vi "AlliGator Save IRFs & Fit Data (Map) HDF5 File v0.4.vi"(0 "File Path":path, 5 "IRFs & Fit Data Map v2":T12 {"Fit Options: Decay Preprocessing Parameters"."# Folds" min=1}, 7 "Decay Fit Options & Parameters":T1 {"Fit Options"."Offset Resolution" min=0.0; "Fit Options"."Period" min=0.0; "Fit Options"."Min Decay Percentile" min=0.0 max=1.0; "Fit Options"."Max Decay Percentile" min=0.0 max=100.0; "Fit Parameter Constraints"."Max Value" format="%#.3g"; "Fit Parameter Constraints"."Min Value" format="%#.3g"}, 9 "Software + Version":string, 11 "Error In":errorcluster, 12 "[Multiple Decays Fit Parameters SDV]":dbl[][](array[numeric])) -> (4 "File Path out":path, 14 "Time (s)":dbl, 15 "Error Out":errorcluster)   [LabVIEW 2021, in "AlliGator Decay Fit Parameter Map.lvlib"]
doc: "Saves Decay Fit Parameter Map and associated metadata to an HDF5 file."
uses:
  AlliGator Decay Fit Parameter Map.lvlib
  AlliGator IRFs & Fit Data v2.ctl
  Fits/IRF(X)PSED/Decay Fit Parameters & Derived Quantities List v2.ctl
  Decay Analysis/Decay Preprocessing/AlliGator Decay Preprocessing Parameters.ctl
  Graphs/XY Graph/XY Graph Plot Shift Parameters.ctl
  Graphs/XY Graph/XY Graph Plot Shift Method.ctl
  AlliGator Decay Fit Options & Parameters v2.ctl
  Fits/IRF(X)PSED/Decay Fit Options v2.ctl
  Fits/Decay Convolution/Decay Model.ctl
  Fits/Residual Type.ctl
  Fits/IRF(X)PSED/Fit Weights Type.ctl
  Fits/Non-linear Fitting Method v2.ctl
  Fits/Fit Calculation Method.ctl
  Fits/Non-linear Fitting Algorithm.ctl
  Decay Analysis/Decay Fit/AlliGator Decay Fit Parameter Constraints 2.ctl
  Fits/IRF(X)PSED/Decay Fit Parameters In List.ctl
  Fits/IRF(X)PSED/MLE Baseline Offset Type.ctl
  <vilib>/addons/h5labview2/file/H5Fmode.ctl
  Globals, Variables, Constants/AlliGator Variables List.ctl
  <vilib>/addons/h5labview2/base/lib_path.vi
  <vilib>/addons/h5labview2/base/H5Equery.vi
  Variant/Variant to Data/Variant to String.vi
  <vilib>/addons/h5labview2/dataset/H5Dwrite.llb/H5Dwrite.xnode
  <vilib>/addons/h5labview2/base/hid_t.ctl
  <vilib>/addons/h5labview2/file/H5F.lvlib
  <vilib>/addons/h5labview2/group/H5G.lvlib
  Time/Time.lvlib
  Utilities/Utilities.lvlib
  Strings/Strings.lvlib
  Globals, Variables, Constants/AlliGator Globals, Variables & Constants.lvlib
  Variant/Variant to Data/Variant to Data.lvlib
  Fits/Fits.lvlib
  Graphs/XY Graph/XY Graph Add-Ons.lvlib
  Decay Analysis/Decay Preprocessing/AlliGator Decay Preprocessing.lvlib
  Decay Analysis/Decay Fit/AlliGator Decay Fit.lvlib
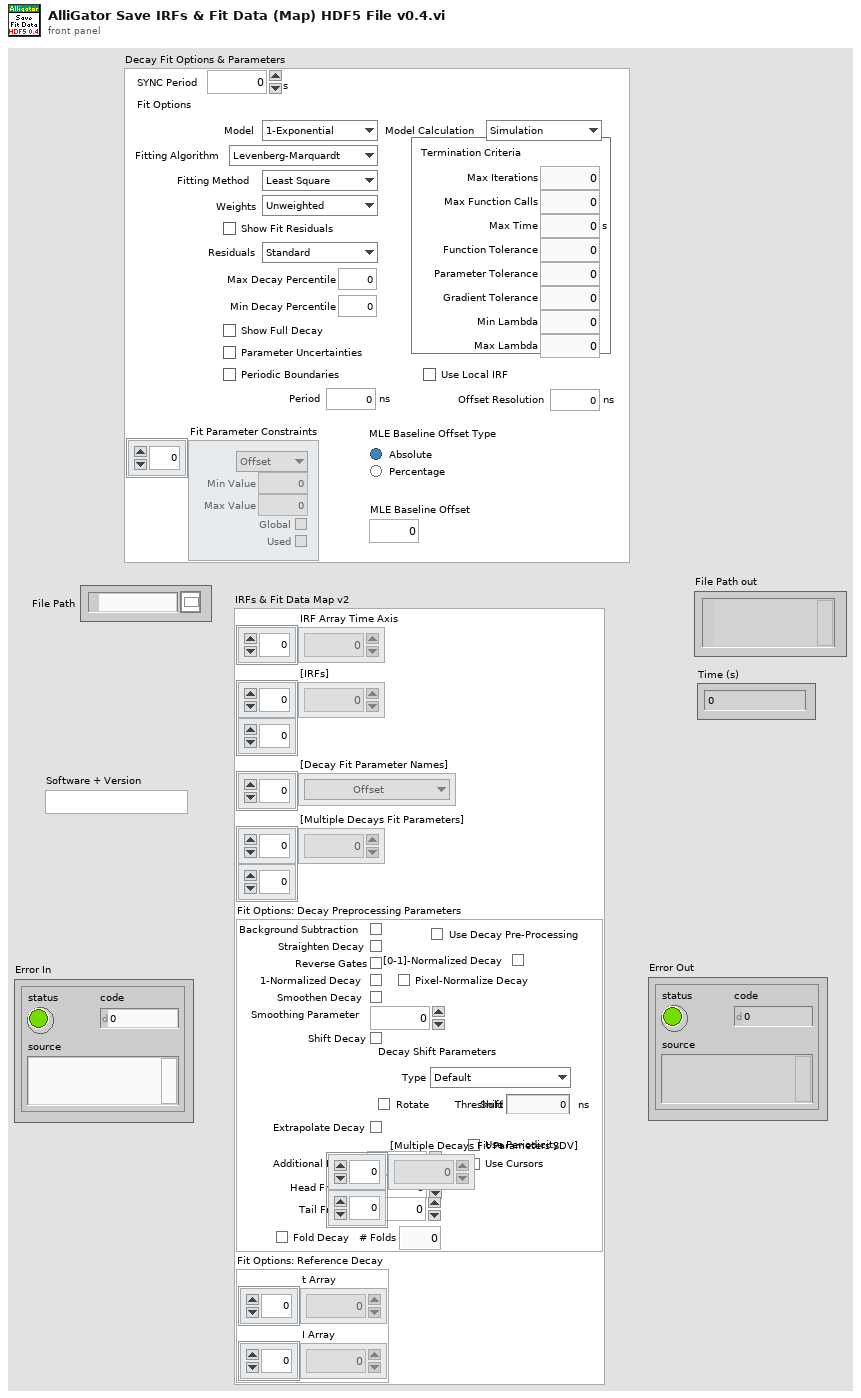
[diagram p1: front panel]
types:
  T1 = typedef "AlliGator Decay Fit Parameter Map.lvlib/AlliGator Decay Fit Options & Parameters v2.ctl" = cluster{"SYNC Period":dbl[unit], "Fit Options":T2, "Fit Parameter Constraints":T9[], "MLE Baseline Offset":dbl, "MLE Baseline Offset Type":T11}
  T2 = typedef "Fits.lvlib/Decay Fit Options v2.ctl" = cluster{"Show Fit Residuals":bool, "Fit Model":T3, "Residual Type":T4, "Max Decay Percentile":dbl, "Min Decay Percentile":dbl, "Show Full Decay":bool, "Weights":T5, "Fitting Method":T6, "Compute Parameter Uncertainties":bool, "Periodic Boundaries":bool, "Model Calculation":T7, "Period":dbl[unit], "Termination Criteria":cluster{"Max Iterations":i32, "Max Function Calls":i32, "Max Time":dbl[unit], "Function Tolerance":dbl, "Parameter Tolerance":dbl, "Gradient Tolerance":dbl, "Min Lambda":dbl, "Max Lambda":dbl, "Initial Tick Count":u32}, "Offset Resolution":dbl[unit], "Use Local IRF":bool, "Fitting Algorithm":T8}
  T3 = typedef "Fits.lvlib/Decay Model.ctl" = enum16{"1-Exponential", "2-Exponentials"}
  T4 = typedef "Fits.lvlib/Residual Type.ctl" = enum16{"Standard", "Normalized", "Reduced"}
  T5 = typedef "Fits.lvlib/Fit Weights Type.ctl" = enum16{"Unweighted", "1/Variance", "Best of All"}
  T6 = typedef "Fits.lvlib/Non-linear Fitting Method v2.ctl" = enum16{"Least Square", "Least Absolute Residual", "Bisquare", "MLE", "-", "Best of All"}
  T7 = typedef "Fits.lvlib/Fit Calculation Method.ctl" = enum16{"Simulation", "Convolution", "Integration"}
  T8 = typedef "Fits.lvlib/Non-linear Fitting Algorithm.ctl" = enum16{"Levenberg-Marquardt", "Trust-Region Dogleg"}
  T9 = typedef "AlliGator Decay Fit.lvlib/AlliGator Decay Fit Parameter Constraints 2.ctl" = cluster{"Fit Parameter":T10, "Min Value":dbl, "Max Value":dbl, "Global":bool, "Used":bool}
  T10 = typedef "Fits.lvlib/Decay Fit Parameters In List.ctl" = enum16{"Offset", "Baseline", "A_1", "tau_1", "A_2", "tau_2"}
  T11 = typedef "Fits.lvlib/MLE Baseline Offset Type.ctl" = enum32{"Absolute", "Percentage"}
  T12 = typedef "AlliGator Decay Fit Parameter Map.lvlib/AlliGator IRFs & Fit Data v2.ctl" = cluster{"IRF Array Time Axis":dbl[], "[IRFs]":dbl[][], "[Decay Fit Parameter Names]":T13[], "[Multiple Decays Fit Parameters]":dbl[][], "Fit Options: Decay Preprocessing Parameters":T14, "Fit Options: Reference Decay":cluster{"t Array":dbl[], "I Array":dbl[]}}
  T13 = typedef "Fits.lvlib/Decay Fit Parameters & Derived Quantities List v2.ctl" = enum16{"Offset", "Baseline", "A_1", "tau_1", "A_2", "tau_2", "<tau>_a", "f1_a", "f2_a", "<tau>_i", "f1_i", "f2_i", "-", "R^2", "Chi^2"}
  T14 = typedef "AlliGator Decay Preprocessing.lvlib/AlliGator Decay Preprocessing Parameters.ctl" = cluster{"Background Subtraction":bool, "Straighten Decay":bool, "Reverse Gates":bool, "1-Normalized Decay":bool, "Smoothen Decay":bool, "Smoothing Parameter":dbl, "Shift Decay":bool, "Decay Shift Parameters":T15, "Extrapolate Decay":bool, "Additional Points":u32, "Head Fraction":dbl, "Pixel-Normalize Decay":bool, "Use Periodicity":bool, "Use Cursors":bool, "Tail Fraction":dbl, "Use Decay Pre-Processing":bool, "Fold Decay":bool, "# Folds":u32, "[0-1]-Normalized Decay":bool}
  T15 = typedef "XY Graph Add-Ons.lvlib/XY Graph Plot Shift Parameters.ctl" = cluster{"Type":T16, "Shift":dbl[unit], "Threshold":dbl, "Rotate":bool}
  T16 = typedef "XY Graph Add-Ons.lvlib/XY Graph Plot Shift Method.ctl" = enum16{"Default", "CFD", "Threshold", "Cross-Correlation"}
  T17 = typedef "AlliGator Globals, Variables & Constants.lvlib/AlliGator Variables List.ctl" = enum16{"---- GUI ----", "GUI:Initialization Status", "GUI:State Indicators Refnum", "GUI:Original AlliGator Menu Items", "GUI:Current Action Loop State", "GUI:Script in progress", "GUI:Playback", "GUI:Loop Playback", "GUI:Search ROI Used", "GUI:Search ROI", "Decay Graph Max Legend Size", "Intensity Graph Max Legend Size", "Decay Statistics Graph Max Legend Size", "Phasor Graph Max Legend Size", "Phasor Ratio Graph Max Legend Size", "Lifetime Graph Max Legend Size", "---- Files ----", "Files:Export Dataset Frames as Individual Files", "Files:Show Batch Export Help Balloons", "Files:Frames in Dataset", "Files:ptu File Frame Start Indices", "Files:Current Frame in Dataset", "Files:Current Frame Timestamp", "Files:Dataset Loaded", "Files:Dataset Metadata", "Files:Dataset Channel", "Files:Dataset Data Description", "Files:Background Dataset Metadata", "Files:Background Dataset Channel", "Files:Background Dataset Data Description", "Files:Background File Subtraction", "Files:Background File Path", "Files:Background File Pile-up Correction", "Files:Background File Pixel Well Capacity", "Files:Background File Scaling Factor", "Files:Current Dataset Load Settings", "Files:Dataset Path", "Files:ICCD-specific Information", "Files:Macrotime Gate Separation", "------ Python Plugins ------", "Python Plugins:Information", "Python Plugins:Python Session", "Python Plugins:Valid Python Session?", "---- Source Image ----", "Source Image:ROIs", "Source Image:Current ROI", "Source Image:ROI Event Refnum", "X_Source Image Display Range", "X_Source Image Palette Information", "X_Type of Displayed Image", "X_Time Gate Slider", "Source Image:Palette List", "Source Image:Scale", "Source Image:ROI Overlay Color", "Source Image:Overlay to Erase", "Source Image:Is Displayed Image Accumulated", "Source Image:White Light Image Modified", "Source Image:Mask Image Modified", "---- Image Profile Window ----", "Image Profile:Window Event Refnum", "Image Profile:IntensityType", "Image Profile:Intensity Average Type", "Image Profile:Intensity-weighted SDV", "Image Profile:Box Profile Type", "Image Profile:Window Open", "Image Profile:Plotted Fit Parameter", "------ Phasor Graph -------", "Phasor Graph:Show Line", "---- Phasor Plot ---", "Phasor Plot:Parameters Changed", "Phasor Plot:FLI Dataset Modified since last Calculation", "Phasor Harmonics Data", "Selected Phasor Harmonics", "Phasor Harmonic Manager Event Refnum", "Phasor Plot:ROIs", "Phasor Plot:Current ROI", "Phasor Plot:ROI Event Refnum", "Phasor Plot:Image Reference Points", "Phasor Plot:Computed", "Phasor Plot:Palette Information", "Phasor Plot:Palette List", "Phasor Plot:Phasor Ratio Palette Information", "Phasor Plot:Phasor Ratio Palette List", "Phasor Plot:Image Scale", "Phasor Plot:Image Overlay to Erase", "Phasor Plot:Image Elements to Update", "Phasor Plot:Current Calculation Parameters", "Phasor Plot:Current Calibration Options", "Phasor Plot:Reset Cumulated Phasor Plot", "Phasor Plot:Reference 1", "Phasor Plot:Lifetime Reference 1", "Phasor Plot:Reference 1 Frequency", "Phasor Plot:Reference 2", "Phasor Plot:Lifetime Reference 2", "Phasor Plot:Reference 2 Frequency", "---- Decay Analysis ----", "Number of Selected Decays to Fit", "LS Fit Results", "LAR Fit Results", "BS Fit Results", "Last Decay Max - Min", "Best Fit Parameters", "Best Fit Parameter Names", "Actual Size X", "Actual Size Y", "Binning X", "Binning Y", "Actual # Gates", "Dataset Number", "Gates to...", "Gates Skipped", "Gates to keep", "Gate Step", "Gate Separation", "Reversed Gates", "Pile-up Correction", "Pixel Well Capacity", "Background Subtracted", "Background Subtraction Method", "Background Definition Range", "Background File (deprecated)", "Number of Dataset Accumulated", "Array of Accumulated Dataset Paths", "Do Averaged Datasets", "Destination File Path", "Process Plot Target", "Use 1/D as Phasor Frequency", "---- Decay Fit Parameter Map -----", "Decay Fit Parameter Map:Palette Information", "Decay Fit Parameter Map:Palette List", "---- Parameter Map ----", "Parameter Map:Palette Information", "Parameter Map:Palette List", "------- Local Decay Window ---------", "Local Decay Graph Window:Event Refnum", "Local Decay Graph Window:Use normalized IRF for convolution", "----- Miscellaneous ----", "Misc:Skippable Dialog Windows Status"}
  T18 = typedef "H5F.lvlib/H5Fmode.ctl" = enum16{"read-only", "read-write", "overwrite", "create new", "open or create"}
  T19 = typedef "hid_t.ctl" = i64
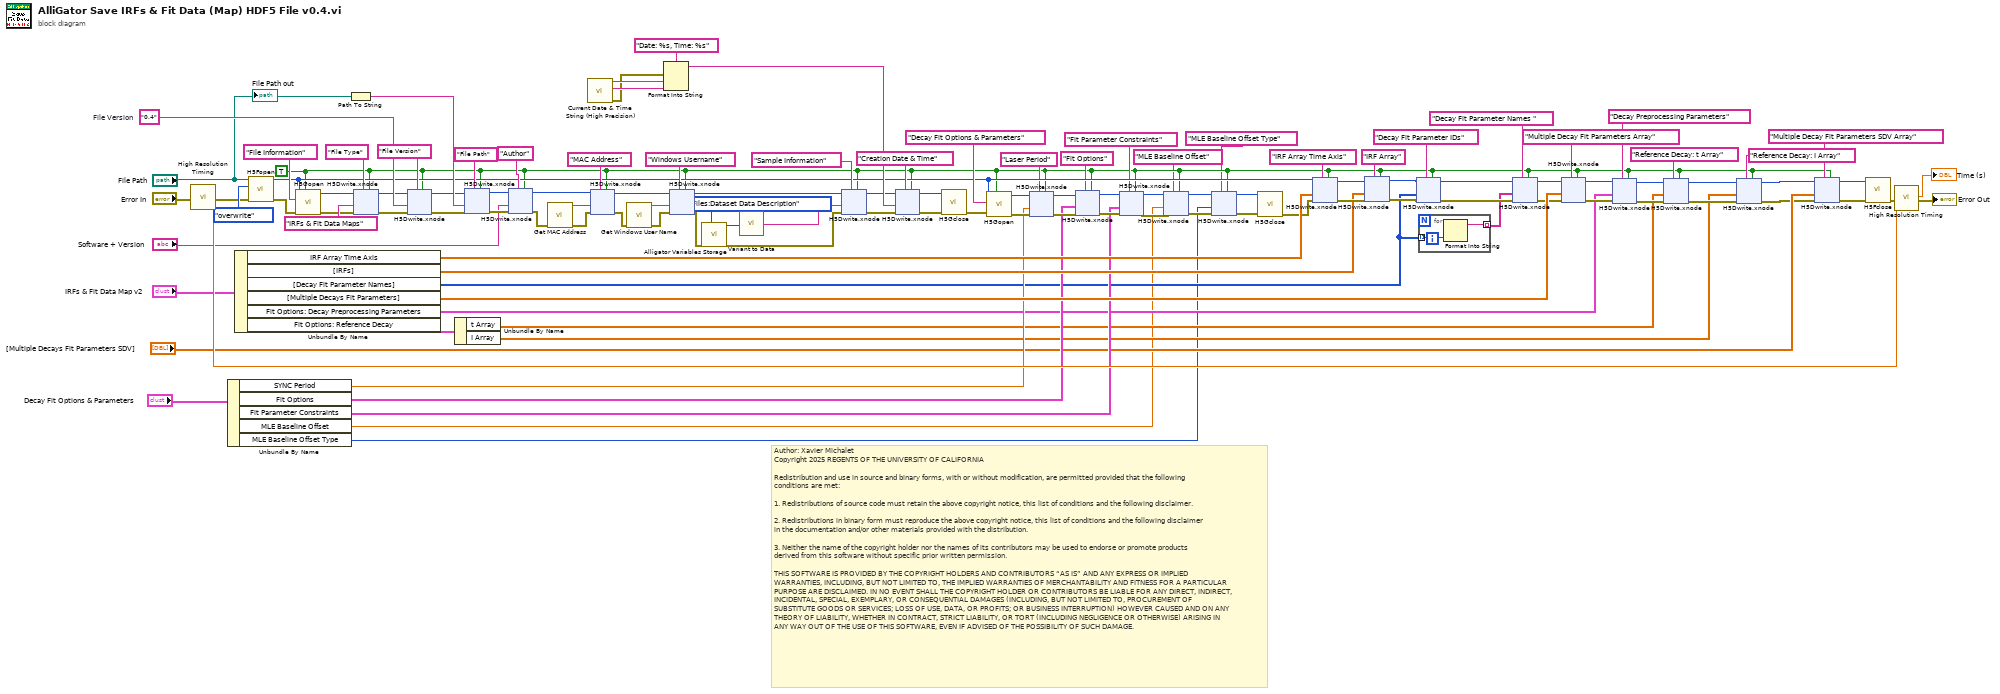
[diagram p0: block diagram]
diagram:
  w110 = "0.4"  # File Version
  w5 = TRUE ("replace? (F)")
  # "Author: Xavier Michalet\nCopyright 2025 REGENTS OF THE UNIVERSITY OF CALIFORNIA\n\nRedistribution and use in source and binary forms, with or without modification, are permitted provided that the following conditions are met:\n\n1. Redistributions of source code must retain the above copyright notice, this list of conditions and the following disclaimer.\n\n2. Redistributions in binary form must reproduce the above copyright notice, this list of conditions and the following disclaimer in the documentation and/or other materials provided with the distribution.\n\n3. Neither the name of the copyright holder nor the names of its contributors may be used to endorse or promote products derived from this software without specific prior written permission.\n\nTHIS SOFTWARE IS PROVIDED BY THE COPYRIGHT HOLDERS AND CONTRIBUTORS “AS IS” AND ANY EXPRESS OR IMPLIED WARRANTIES, INCLUDING, BUT NOT LIMITED TO, THE IMPLIED WARRANTIES OF MERCHANTABILITY AND FITNESS FOR A PARTICULAR PURPOSE ARE DISCLAIMED. IN NO EVENT SHALL THE COPYRIGHT HOLDER OR CONTRIBUTORS BE LIABLE FOR ANY DIRECT, INDIRECT, INCIDENTAL, SPECIAL, EXEMPLARY, OR CONSEQUENTIAL DAMAGES (INCLUDING, BUT NOT LIMITED TO, PROCUREMENT OF SUBSTITUTE GOODS OR SERVICES; LOSS OF USE, DATA, OR PROFITS; OR BUSINESS INTERRUPTION) HOWEVER CAUSED AND ON ANY THEORY OF LIABILITY, WHETHER IN CONTRACT, STRICT LIABILITY, OR TORT (INCLUDING NEGLIGENCE OR OTHERWISE) ARISING IN ANY WAY OUT OF THE USE OF THIS SOFTWARE, EVEN IF ADVISED OF THE POSSIBILITY OF SUCH DAMAGE."
  n1 = call "High Resolution Timing.vi"("Error In"="Error In") -> ("elapsed (relative) seconds"=w113:dbl, "Error Out"=w115:errorcluster)  [unwired: 16 in, 1 out]
  n2 = Unbundle By Name("Decay Fit Options & Parameters") -> ("SYNC Period"=w47:dbl[unit], "Fit Options"=w44:T2, "Fit Parameter Constraints"=w43:T9[], "MLE Baseline Offset"=w3:dbl, "MLE Baseline Offset Type"=w2:T11)
  n3 = Unbundle By Name("IRFs & Fit Data Map v2") -> ("IRF Array Time Axis"=w69:dbl[], "[IRFs]"=w68:dbl[][], "[Decay Fit Parameter Names]"=w29:T13[], "[Multiple Decays Fit Parameters]"=w63:dbl[][], "Fit Options: Decay Preprocessing Parameters"=w20:T14, "Fit Options: Reference Decay"=w19:cluster{"t Array":dbl[], "I Array":dbl[]})
  n4 = call <vilib>:"H5Fopen.vi"("error in (no error)"=w115, "mode (read-only)"=H5Fmode."overwrite", "path"="File Path") -> ("error out"=w117:errorcluster, "ref out"=w53:T19)  [unwired: 7 in]
  n5 = call <vilib>:"H5Gopen.vi"("create? (F)"=w5, "error in (no error)"=w117, "name"="File Information", "ref in"=w53) -> ("error out"=w105:errorcluster, "group out"=w102:T19)  [unwired: 6 in]
  n6 = Path To String(path="File Path") -> (string=w89:string)
  n7 = xnode "H5Dwrite.xnode"("replace? (F)"=w5, "dataset name"="File Type", "error in (no error)"=w105, "data"="IRFs & Fit Data Maps" ("dataset name"), "ref in"=w102) -> ("error out"=w61:errorcluster, "ref out"=w62:i64)  [unwired: 2 in, 1 out]
  n8 = xnode "H5Dwrite.xnode"("replace? (F)"=w5, "dataset name"="File Version", "error in (no error)"=w61, "data"=w110, "ref in"=w62) -> ("error out"=w60:errorcluster, "ref out"=w59:T19)  [unwired: 2 in, 1 out]
  n9 = Unbundle By Name(w19) -> ("t Array"=w18:dbl[], "I Array"=w12:dbl[])
  n10 = xnode "H5Dwrite.xnode"("replace? (F)"=w5, "dataset name"="File Path", "error in (no error)"=w60, "data"=w89, "ref in"=w59) -> ("error out"=w99:errorcluster, "ref out"=w100:T19)  [unwired: 2 in, 1 out]
  n11 = xnode "H5Dwrite.xnode"("replace? (F)"=w5, "dataset name"="Author", "error in (no error)"=w99, "data"="Software + Version", "ref in"=w100) -> ("error out"=w37:errorcluster, "ref out"=w97:T19)  [unwired: 2 in, 1 out]
  n12 = call "Get MAC Address.vi"("Error In"=w37) -> ("Error Out"=w36:errorcluster, "MAC address"=w94:string)  [unwired: 9 in]
  n13 = call "Current Date & Time String (High Precision).vi"() -> ("Error Out"=w86:errorcluster, "time string"=w87:string, "date string"=w88:string)  [unwired: 8 in, 1 out]
  n14 = xnode "H5Dwrite.xnode"("replace? (F)"=w5, "dataset name"="MAC Address", "error in (no error)"=w36, "data"=w94, "ref in"=w97) -> ("error out"=w35:errorcluster, "ref out"=w96:T19)  [unwired: 2 in, 1 out]
  n15 = call "Get Windows User Name.vi"("Error In"=w35) -> ("Error Out"=w34:errorcluster, "User Name"=w92:string)  [unwired: 9 in]
  n16 = Format Into String(format string="Date: %s, Time: %s", error in=w86, w88, w87) -> (resulting string=w83:string)  [unwired: 1 in, 1 out]
  n17 = xnode "H5Dwrite.xnode"("replace? (F)"=w5, "dataset name"="Windows Username", "error in (no error)"=w34, "data"=w92, "ref in"=w96) -> ("error out"=w75:errorcluster, "ref out"=w81:T19)  [unwired: 2 in, 1 out]
  n18 = call "Alligator Variables Storage.vi"("AlliGator Variable"=AlliGator_Variables_List."Files:Dataset Data Description" ("Alligator Variable"), "Error In"=w75) -> ("Error Out"=w74:errorcluster, "Data out"=w77:variant)  [unwired: 7 in, 1 out]
  n19 = call-poly "Variant to Data.vi"("Variant"=w77) -> ("String"=w76:string)  [unwired: 8 in]
  n20 = xnode "H5Dwrite.xnode"("replace? (F)"=w5, "dataset name"="Sample Information" ("name"), "error in (no error)"=w74, "data"=w76, "ref in"=w81) -> ("error out"=w82:errorcluster, "ref out"=w80:T19)  [unwired: 2 in, 1 out]
  n21 = xnode "H5Dwrite.xnode"("replace? (F)"=w5, "dataset name"="Creation Date & Time", "error in (no error)"=w82, "data"=w83, "ref in"=w80) -> ("error out"=w71:errorcluster, "ref out"=w72:T19)  [unwired: 2 in, 1 out]
  n22 = call <vilib>:"H5Gclose.vi"("error in (no error)"=w71, "group in"=w72) -> ("error out"=w58:errorcluster)  [unwired: 9 in]
  n23 = call <vilib>:"H5Gopen.vi"("create? (F)"=w5, "error in (no error)"=w58, "name"="Decay Fit Options & Parameters" ("dataset name"), "ref in"=w53) -> ("error out"=w56:errorcluster, "group out"=w55:T19)  [unwired: 6 in]
  n24 = xnode "H5Dwrite.xnode"("replace? (F)"=w5, "dataset name"="Laser Period", "error in (no error)"=w56, "data"=w47, "ref in"=w55) -> ("error out"=w52:errorcluster, "ref out"=w50:T19)  [unwired: 2 in, 1 out]
  n25 = xnode "H5Dwrite.xnode"("replace? (F)"=w5, "dataset name"="Fit Options", "error in (no error)"=w52, "data"=w44, "ref in"=w50) -> ("error out"=w51:errorcluster, "ref out"=w49:i64)  [unwired: 2 in, 1 out]
  n26 = xnode "H5Dwrite.xnode"("replace? (F)"=w5, "dataset name"="Fit Parameter Constraints", "error in (no error)"=w51, "data"=w43, "ref in"=w49) -> ("error out"=w11:errorcluster, "ref out"=w10:i64)  [unwired: 2 in, 1 out]
  n27 = xnode "H5Dwrite.xnode"("replace? (F)"=w5, "dataset name"="MLE Baseline Offset", "error in (no error)"=w11, "data"=w3, "ref in"=w10) -> ("error out"=w9:errorcluster, "ref out"=w7:i64)  [unwired: 2 in, 1 out]
  n28 = xnode "H5Dwrite.xnode"("replace? (F)"=w5, "dataset name"="MLE Baseline Offset Type", "error in (no error)"=w9, "data"=w2, "ref in"=w7) -> ("error out"=w8:errorcluster, "ref out"=w6:i64)  [unwired: 2 in, 1 out]
  n29 = call <vilib>:"H5Gclose.vi"("error in (no error)"=w8, "group in"=w6) -> ("error out"=w54:errorcluster)  [unwired: 9 in]
  n30 = xnode "H5Dwrite.xnode"("replace? (F)"=w5, "dataset name"="IRF Array Time Axis", "error in (no error)"=w54, "data"=w69, "ref in"=w53) -> ("error out"=w108:errorcluster, "ref out"=w109:T19)  [unwired: 2 in, 1 out]
  n31 = xnode "H5Dwrite.xnode"("replace? (F)"=w5, "dataset name"="IRF Array", "error in (no error)"=w108, "data"=w68, "ref in"=w109) -> ("error out"=w66:errorcluster, "ref out"=w67:T19)  [unwired: 2 in, 1 out]
  n32 = xnode "H5Dwrite.xnode"("replace? (F)"=w5, "dataset name"="Decay Fit Parameter IDs" ("name"), "error in (no error)"=w66, "data"=w29, "ref in"=w67) -> ("error out"=w32:errorcluster, "ref out"=w33:i64)  [unwired: 2 in, 1 out]
  n33 = for {
    tunnel: w29 -> [w121] mode=indexing
    tunnel: [w120] -> w28 mode=indexing
    n34 = Format Into String(w121) -> (resulting string=w120:string)  [unwired: 3 in, 1 out]
  }
  n35 = xnode "H5Dwrite.xnode"("replace? (F)"=w5, "dataset name"="Decay Fit Parameter Names " ("name"), "error in (no error)"=w32, "data"=w28, "ref in"=w33) -> ("error out"=w31:errorcluster, "ref out"=w30:T19)  [unwired: 2 in, 1 out]
  n36 = xnode "H5Dwrite.xnode"("replace? (F)"=w5, "dataset name"="Multiple Decay Fit Parameters Array" ("name"), "error in (no error)"=w31, "data"=w63, "ref in"=w30) -> ("error out"=w24:errorcluster, "ref out"=w26:T19)  [unwired: 2 in, 1 out]
  n37 = xnode "H5Dwrite.xnode"("replace? (F)"=w5, "dataset name"="Decay Preprocessing Parameters" ("name"), "error in (no error)"=w24, "data"=w20, "ref in"=w26) -> ("error out"=w23:errorcluster, "ref out"=w25:i64)  [unwired: 2 in, 1 out]
  n38 = xnode "H5Dwrite.xnode"("replace? (F)"=w5, "dataset name"="Reference Decay: t Array" ("name"), "error in (no error)"=w23, "data"=w18, "ref in"=w25) -> ("error out"=w17:errorcluster, "ref out"=w16:T19)  [unwired: 2 in, 1 out]
  n39 = xnode "H5Dwrite.xnode"("replace? (F)"=w5, "dataset name"="Reference Decay: I Array" ("name"), "error in (no error)"=w17, "data"=w12, "ref in"=w16) -> ("error out"=w14:errorcluster, "ref out"=w15:T19)  [unwired: 2 in, 1 out]
  n40 = xnode "H5Dwrite.xnode"("replace? (F)"=w5, "dataset name"="Multiple Decay Fit Parameters SDV Array" ("name"), "error in (no error)"=w14, "data"="[Multiple Decays Fit Parameters SDV]", "ref in"=w15) -> ("error out"=w40:errorcluster, "ref out"=w41:T19)  [unwired: 2 in, 1 out]
  n41 = call <vilib>:"H5Fclose.vi"("error in (no error)"=w40, "ref"=w41) -> ("error out"=w119:errorcluster)  [unwired: 9 in]
  n42 = call "High Resolution Timing.vi"("relative seconds (NaN)"=w113, "Error In"=w119) -> ("elapsed (relative) seconds"=→"Time (s)":dbl, "Error Out"=→"Error Out":errorcluster)  [unwired: 15 in, 1 out]
  "File Path out" <- "File Path"
